vi "StopSignal-Prototype.vi"() -> ()   [LabVIEW 2017, in "StopSignal.lvlib"]
uses:
  StopSignal.lvlib
panel:
  out "reason #4":string
  out "reason #1":string
  out "reason #2":string
  out "reason #3":string
  out "current time":timestamp
  in  "stop":bool
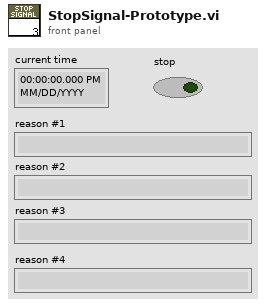
[diagram p1: front panel]
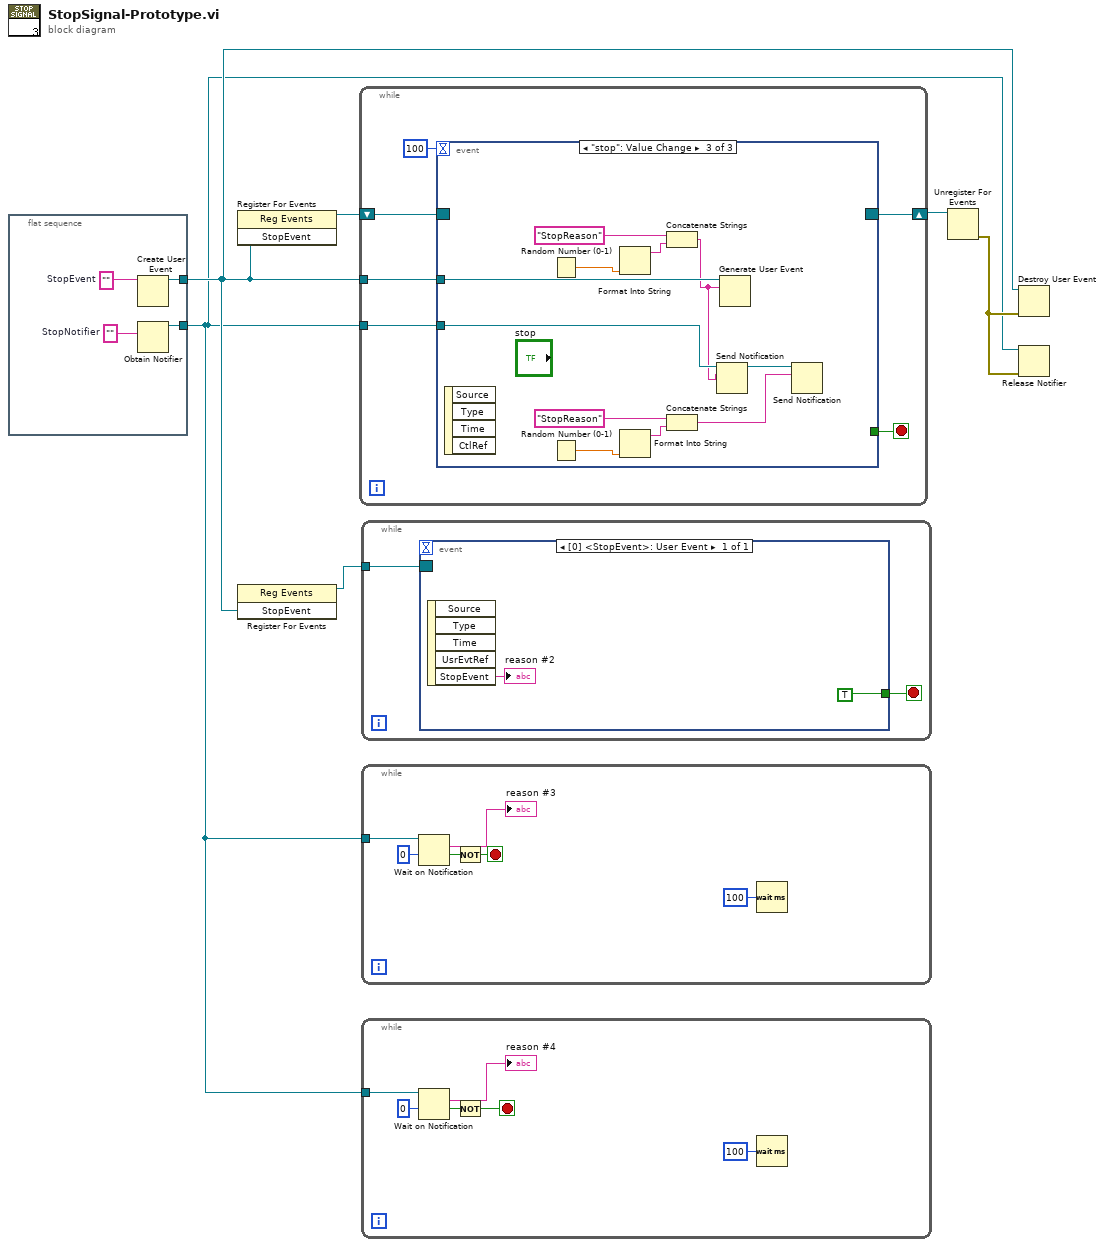
[diagram p0: block diagram]
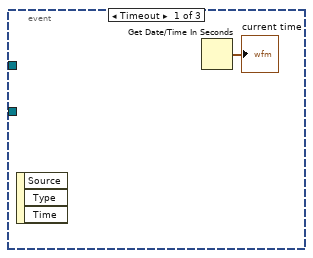
[diagram p2: hidden frame]
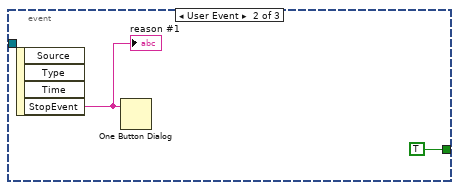
[diagram p3: hidden frame]
diagram:
  n1 = flat-sequence {
    tunnel: [w8] -> w3
    tunnel: [w7] -> w1
    frame #0 {
      w9 = ""  # StopNotifier
      w10 = ""  # StopEvent
      n2 = Create User Event(user event datatype=w10) -> (user event=w8:refnum<user-event>)  [unwired: 1 in, 1 out]
      n3 = Obtain Notifier(notification data type=w9) -> (notifier out=w7:refnum<notifier>)  [unwired: 3 in, 2 out]
    }
  }
  n4 = register-events(w3) -> (reference out=w6:refnum<event-registration>)  [unwired: 2 in, 1 out]
  n5 = register-events(w3) -> (reference out=w4:refnum<event-registration>)  [unwired: 2 in, 1 out]
  n6 = while {
    tunnel: w3 -> [w15]
    shift-right: [w12] -> w5
    shift-left: w6 -> [w16]
    tunnel: w1 -> [w11]
    stop <- w14 stop-if-true
    n7 = event shown="[2] \"stop\": Value Change" {
      selector: w16 -> [_ _ _]
      dyn-events: [_ _ _] -> w12
      timeout: 100 -> [_ _ _]
      tunnel: w15 -> [_ _ w30]
      tunnel: [_ TRUE _] -> w14
      tunnel: w11 -> [_ _ w28]
      event Timeout {
        n8 = event-data() -> ()  [unwired: 1 in, 3 out]
        n9 = Get Date/Time In Seconds() -> (seconds since 1Jan1904=→"current time":timestamp)
      }
      event User Event {
        n10 = event-data() -> ("StopEvent"=w18:string)  [unwired: 1 in, 3 out]
        "reason #1" <- w18
        n11 = One Button Dialog(message=w18) -> ()  [unwired: 1 in, 1 out]
      }
      event "stop": Value Change {
        n12 = event-data() -> ()  [unwired: 1 in, 4 out]
        n13 = Random Number (0-1)() -> (number: 0 to 1=w27:dbl)
        n14 = Random Number (0-1)() -> (number: 0 to 1=w23:dbl)
        n15 = Format Into String(w27) -> (resulting string=w26:string)  [unwired: 3 in, 1 out]
        n16 = Format Into String(w23) -> (resulting string=w24:string)  [unwired: 3 in, 1 out]
        n17 = Concatenate Strings("StopReason" ("event data"), w26) -> (w25:string)
        n18 = Concatenate Strings("StopReason" ("event data"), w24) -> (w20:string)
        n19 = Send Notification(notification=w25, notifier=w28) -> (notifier out=w21:refnum<notifier>)  [unwired: 1 in, 1 out]
        n20 = Generate User Event(user event=w30, event data cluster=w25) -> ()  [unwired: 2 in, 2 out]
        n21 = Send Notification(notification=w20, notifier=w21) -> ()  [unwired: 1 in, 2 out]
      }
    }
  }
  n22 = while {
    tunnel: w4 -> [w32]
    stop <- w31 stop-if-true
    n23 = event shown="[0] <StopEvent>: User Event" {
      selector: w32 -> [_]
      dyn-events: _ -> [_]
      timeout: _ -> [_]
      tunnel: [TRUE] -> w31
      event User Event {
        n24 = event-data() -> ("StopEvent"=→"reason #2":string)  [unwired: 1 in, 4 out]
      }
    }
  }
  n25 = while {
    tunnel: w1 -> [w40]
    stop <- w35 stop-if-true
    n26 = Wait on Notification(notifier=w40, timeout in ms (-1)=0) -> (notification=→"reason #3":string, timed out?=w38:bool)  [unwired: 2 in, 2 out]
    n27 = Not(x=w38) -> (.not. x?=w35:bool)
    n28 = Wait (ms)(milliseconds to wait=u32 100) -> ()  [unwired: 1 out]
  }
  n29 = while {
    tunnel: w1 -> [w46]
    stop <- w41 stop-if-true
    n30 = Wait on Notification(notifier=w46, timeout in ms (-1)=0) -> (notification=→"reason #4":string, timed out?=w44:bool)  [unwired: 2 in, 2 out]
    n31 = Not(x=w44) -> (.not. x?=w41:bool)
    n32 = Wait (ms)(milliseconds to wait=u32 100) -> ()  [unwired: 1 out]
  }
  n33 = Unregister For Events(event registration refnum=w5) -> (error out=w2:errorcluster)  [unwired: 1 in]
  n34 = Destroy User Event(user event=w3, error in=w2) -> ()  [unwired: 1 out]
  n35 = Release Notifier(notifier=w1, error in (no error)=w2) -> ()  [unwired: 1 in, 3 out]
